vi "Remove Unused Channels.vi"(0 "Data in":sgl[][](array[numeric]), 7 "Channel Filter":bool[](array[boolean])) -> (4 "Data out":sgl[][](array[numeric]))   [LabVIEW 2023]
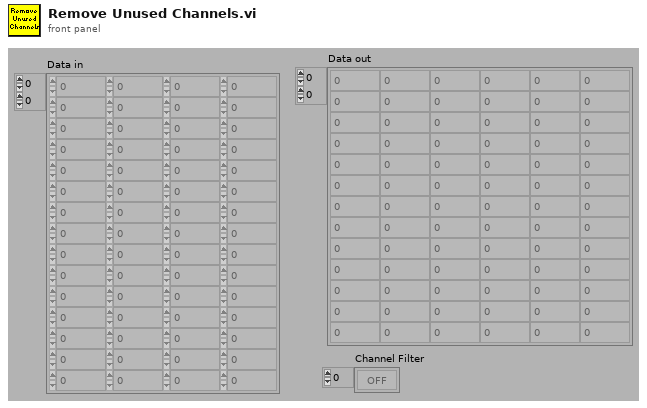
[diagram p1: front panel]
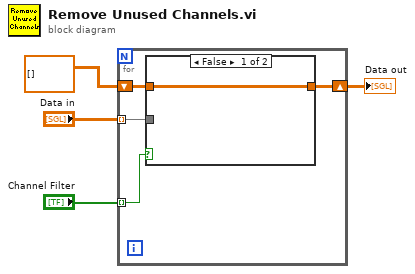
[diagram p0: block diagram]
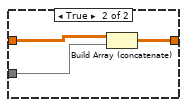
[diagram p2: hidden frame]
diagram:
  n1 = for {
    tunnel: "Data in" -> [w5] mode=indexing
    tunnel: "Channel Filter" -> [w6] mode=indexing
    shift-right: [w8] -> w1
    shift-left: sgl[][] [] ("Data in") -> [w7]
    n2 = case shown="False" w6 {
      tunnel: [w9 w12] -> w8
      tunnel: w7 -> [w9 w11]
      tunnel: w5 -> [_ w10]
      frame False {
      }
      frame True {
        n3 = Build Array (concatenate)(w11, w10) -> (w12:sgl[][])
      }
    }
  }
  "Data out" <- w1
